vi "Configure IQ vs Slot Measurement Timeout.vi"(8 "error in (no error)":errorcluster, 9 "Timeout (1)":i32=1, 10 "Instance (1)":i32=1, 11 "VISA resource name":refnum<visa-resource-name>) -> (0 "error out":errorcluster, 3 "VISA resource name out":refnum<visa-resource-name>)   [LabVIEW 2020, in "Rohde&Schwarz CMXP GPRF.lvlib"]
doc: "Defines a timeout for the measurement.\n\nAttribute:\nRSCMXPGPRF_ATTR_IQ_VS_SLOT_MEASUREMENT_TIMEOUT\n\nRemote-control command:\nCONFigure:GPRF:MEAS<i>:IQVSlot:TOUT"
uses:
  <instrlib>/Rohde&Schwarz CMXP GPRF/Rohde&Schwarz CMXP GPRF.lvlib
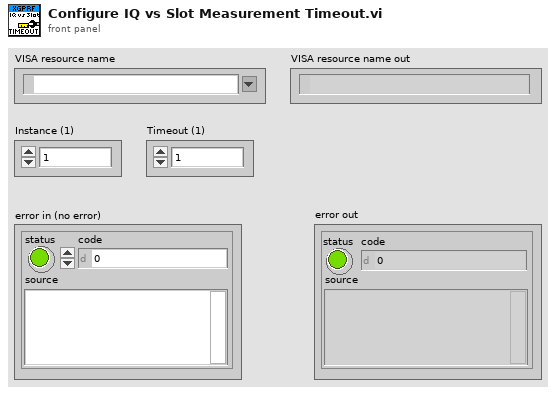
[diagram p1: front panel]
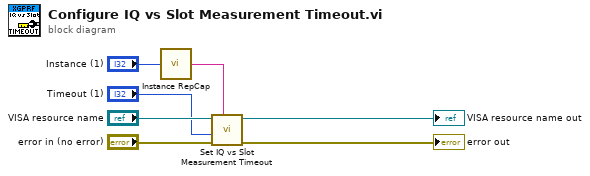
[diagram p0: block diagram]
diagram:
  n1 = call <instrlib>:"Instance RepCap.vi"("Instance in"="Instance (1)") -> ("Instance out"=w6:string)
  n2 = call "Set IQ vs Slot Measurement Timeout"("Repeated Capabilities"=w6, "error in (no error)"="error in (no error)", "IQ vs Slot Measurement Timeout (0.0)"="Timeout (1)", "instrument handle"="VISA resource name") -> ("error out"=→"error out":errorcluster, "instrument handle out"=→"VISA resource name out":refnum<visa-resource-name>)  [unwired: 6 in]
